vi "regEvt.vi"(8 "error in (no error)":errorcluster, 10 "evtReg":string[][](array[string]), 11 "tcpServer in":refnum<class "TcpServer.lvclass">) -> (0 "error out":errorcluster, 3 "tcpServer out":refnum<class "TcpServer.lvclass">)   [LabVIEW 2018, in "TcpServer.lvclass"]
doc: "Inform the TCP Server which events are registered and allowed to be processed. \n\nFor instance,\n\n| compName | evtName |\n| ---------------- | ------------- |\n| Dome | move |"
uses:
  TcpServer.lvclass
  TcpServer.lvclass/TcpServer.ctl
  TcpServerBase/TcpServerBase.lvclass/TcpServerBase.ctl
  TcpServerCmd/TcpServerCmd.lvclass
  home/pcortes/github/ts_labview_tcp_json/src/TcpServerBase/TcpServerBase.lvclass
  TcpServerBase/TcpServerBase.lvclass
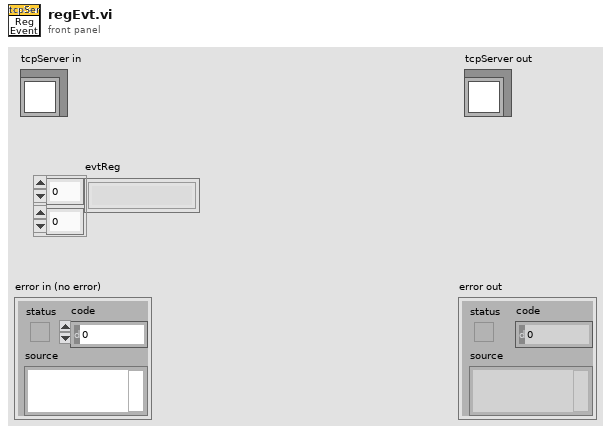
[diagram p1: front panel]
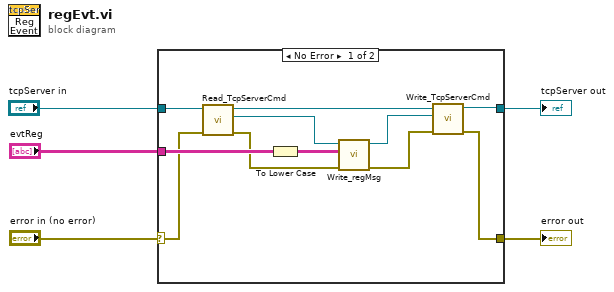
[diagram p0: block diagram]
diagram:
  n1 = case shown="No Error" "error in (no error)" {
    selector: "error in (no error)" -> [w12 w18]
    tunnel: [w6 w18] -> w4
    tunnel: [w10 w17] -> w1
    tunnel: "tcpServer in" -> [w14 w17]
    tunnel: "evtReg" -> [w16 _]
    frame No Error {
      n2 = call "Read_TcpServerCmd.vi"("error in (no error)"=w12, "TcpServer in"=w14) -> ("error out"=w11:errorcluster, "TcpServerCmd.lvclass"=w13:refnum<class "TcpServerCmd.lvclass">, "TcpServer out"=w9:refnum<class "TcpServer.lvclass">)  [unwired: 7 in]
      n3 = To Lower Case(string=w16) -> (all lower case string=w15:string[][])
      n4 = call "Write_regMsg.vi"("error in (no error)"=w11, "regMsg"=w15, "TcpServerBase in"=w13) -> ("error out"=w7:errorcluster, "TcpServerBase out"=w8:refnum<class "TcpServerCmd.lvclass">)  [unwired: 7 in]
      n5 = call "Write_TcpServerCmd.vi"("error in (no error)"=w7, "TcpServerCmd.lvclass"=w8, "TcpServer in"=w9) -> ("error out"=w6:errorcluster, "TcpServer out"=w10:refnum<class "TcpServer.lvclass">)  [unwired: 7 in]
    }
    frame Error {
    }
  }
  "error out" <- w4
  "tcpServer out" <- w1
